vi "Set Attributes.vi"(8 "error in (no error)":errorcluster, 11 "Sequence Dialog in":refnum<class "TestStep Edit Dialog.lvclass">) -> (0 "error out":errorcluster, 3 "Sequence Dialog out":refnum<class "TestStep Edit Dialog.lvclass">)   [LabVIEW 2017, in "TestStep Edit Dialog.lvclass"]
uses:
  TestStep Edit Dialog.lvclass
  D:/Test-executive-builder/Source/Test Executive Builder Dialogs/ITest Executive Builder Dialog/ITest Executive Builder Dialog.lvclass
  ITest Executive Builder Dialog/ITest Executive Builder Dialog.lvclass/ITest Executive Builder Dialog.ctl
  TestStep Edit Dialog.lvclass/TestStep Edit Dialog.ctl
  4517e7d4-0062-47fd-b097-7c0ba10c9864.vi
  039e43ab-2486-4d13-8cf7-732014498f39.vi
  b5a19295-ccfe-4040-b50d-89a8fe728640.vi
  <vilib>/Utility/error.llb/Error Cluster From Error Code.vi
  <vilib>/gpm_packages/@cs/test-executive/Source/Test Executive/ITestExecutive/ITest Executive.lvclass
  ITest Executive Builder Dialog/ITest Executive Builder Dialog.lvclass
  <vilib>/gpm_packages/@cs/test-executive/Source/Test Executive/TestExecutive Ref/TestExecutive Ref.lvclass
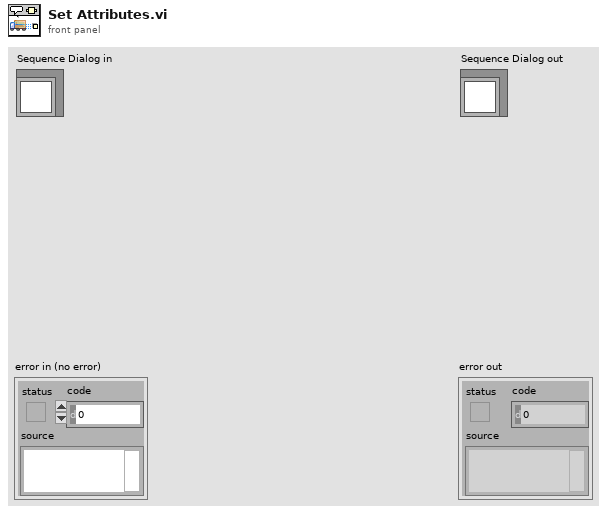
[diagram p1: front panel]
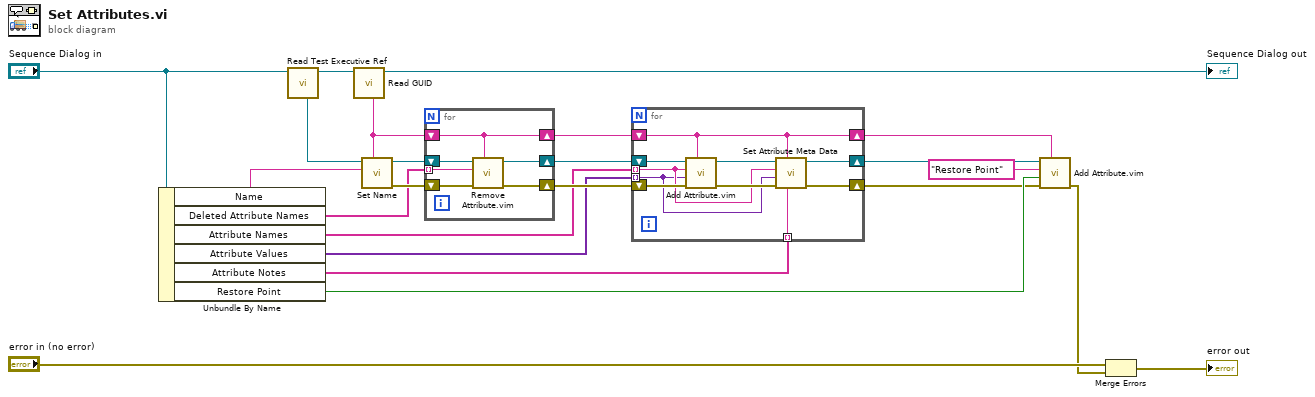
[diagram p0: block diagram]
diagram:
  n1 = Unbundle By Name("Sequence Dialog in") -> ("Name"=w21:string, "Deleted Attribute Names"=w17:string[], "Attribute Names"=w13:string[], "Attribute Values"=w12:variant[], "Attribute Notes"=w6:string[], "Restore Point"=w11:bool)
  n2 = call "Read Test Executive Ref.vi"("ITest Executive Builder Dialog in"="Sequence Dialog in") -> ("ITest Executive Builder Dialog out"=w23:refnum<class "TestStep Edit Dialog.lvclass">, "Test Executive Ref"=w22:refnum<data-value>)  [unwired: 9 in]
  n3 = call "Read GUID.vi"("ITest Executive Builder Dialog in"=w23) -> ("ITest Executive Builder Dialog out"=→"Sequence Dialog out":refnum<class "TestStep Edit Dialog.lvclass">, "GUID"=w19:string)  [unwired: 9 in]
  n4 = call <vilib>:"Set Name.vi"("Unique ID"=w19, "Name"=w21, "Test Executive Ref"=w22) -> ("error out"=w18:errorcluster, "Test Executive Ref out"=w20:refnum<data-value>)  [unwired: 7 in]
  n5 = for {
    shift-right: [w28] -> w14
    shift-left: w19 -> [w28]
    shift-right: [w26] -> w16
    shift-left: w20 -> [w29]
    shift-right: [w25] -> w15
    shift-left: w18 -> [w27]
    tunnel: w17 -> [w24] mode=indexing
    n6 = call "Remove Attribute.vim"("ID"=w28, "error in (no error)"=w27, "Attribute Name"=w24, "Test Executive Ref"=w29) -> ("error out"=w25:errorcluster, "Test Executive Ref out"=w26:refnum<data-value>)  [unwired: 5 in, 1 out]
  }
  n7 = for {
    shift-right: [w36] -> w8
    shift-left: w16 -> [w39]
    shift-right: [w34] -> w7
    shift-left: w15 -> [w38]
    tunnel: w13 -> [w32] mode=indexing
    tunnel: w12 -> [w31] mode=indexing
    shift-right: [w30] -> w9
    shift-left: w14 -> [w30]
    tunnel: w6 -> [w33] mode=indexing
    n8 = call "Add Attribute.vim"("ID"=w30, "error in (no error)"=w38, "Attribute"=w31, "Attribute Name"=w32, "Test Executive Ref"=w39) -> ("error out"=w35:errorcluster, "Test Executive Ref out"=w37:refnum<data-value>)  [unwired: 3 in, 2 out]
    n9 = call <vilib>:"Set Attribute Meta Data.vi"("Meta Data"=w33, "Unique ID"=w30, "error in (no error)"=w35, "Attribute Type"=w31, "Attribute Name"=w32, "Test Executive Ref"=w37) -> ("error out"=w34:errorcluster, "Test Executive Ref out"=w36:refnum<data-value>)  [unwired: 3 in, 1 out]
  }
  n10 = call "Add Attribute.vim"("ID"=w9, "error in (no error)"=w7, "Attribute"=w11, "Attribute Name"="Restore Point", "Test Executive Ref"=w8) -> ("error out"=w2:errorcluster)  [unwired: 3 in, 3 out]
  n11 = Merge Errors("error in (no error)", w2) -> (→"error out":errorcluster)
